vi "Outdent Subsquent Report.vi"(0 "report in":refnum<class "NI_HTML.lvclass">, 7 "level":i32, 11 "error in (no error)":errorcluster) -> (4 "report out":refnum<class "NI_HTML.lvclass">, 15 "error out":errorcluster)   [LabVIEW 2020, in "NI_HTML.lvclass"]
uses:
  <vilib>/Utility/NIReport.llb/HTML/NI_HTML.lvclass
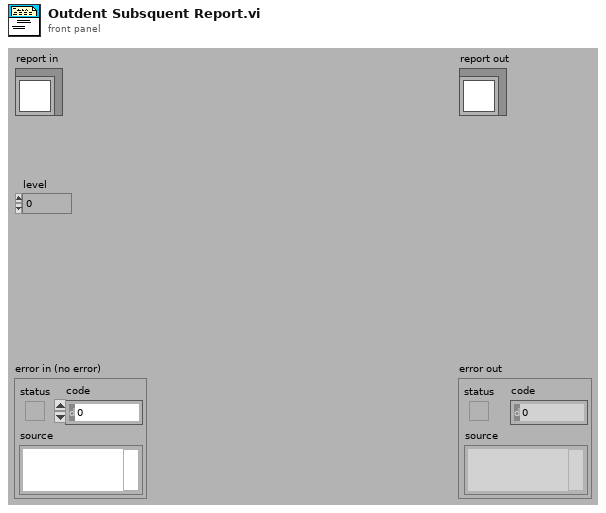
[diagram p1: front panel]
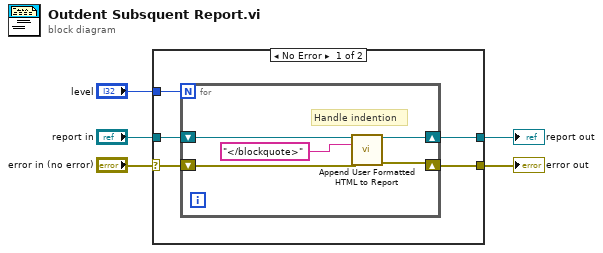
[diagram p0: block diagram]
diagram:
  n1 = case shown="No Error" "error in (no error)" {
    selector: "error in (no error)" -> [w8 w17]
    tunnel: [w7 w17] -> w4
    tunnel: [w9 w16] -> w2
    tunnel: "report in" -> [w10 w16]
    tunnel: "level" -> [w6 _]
    frame No Error {
      n2 = for {
        N: w6 -> [_]
        shift-right: [w14] -> w7
        shift-left: w8 -> [w15]
        shift-right: [w11] -> w9
        shift-left: w10 -> [w12]
        # "Handle indention"
        n3 = call-dynamic "Append User Formatted HTML to Report.vi"("report in"=w12, "HTML text"="</blockquote>" ("text"), "error in (no error)"=w15) -> ("report out"=w11:refnum<class "NI_HTML.lvclass">, "error out"=w14:errorcluster)  [unwired: 11 out]
      }
    }
    frame Error {
    }
  }
  "error out" <- w4
  "report out" <- w2
